vi "InjectionLockServo.vi"() -> ()   [LabVIEW 2020]
panel:
  out "Down times":dbl
  out "Up times":dbl
  out "Currently Output (mA)":dbl
  in  "Initial Output (mA)":dbl
  out "min-max":dbl
  out "min value":dbl
  out "max value":dbl
  in  "?":bool
  in  "Unlock Step\nLength (mA)":dbl
  in  "Semi-lock Step \nLength (mA)":dbl
  in  "Noise Threshold (V)":dbl
  in  "Lock Threshold (V)":dbl
  in  "rate":dbl=10000.0
  in  "milliseconds to wait":u32
  in  "number of samples":i32=100
  out "Waveform Chart":dynamicdata(graph)
  # "Result of Sampling"
  # "Parameters of Feedback"
  # "Parameters of Sampling"
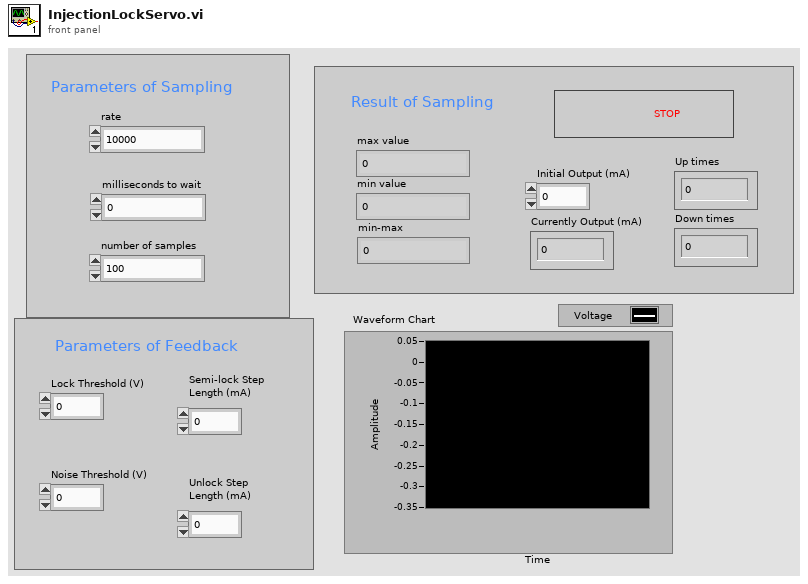
[diagram p1: front panel]
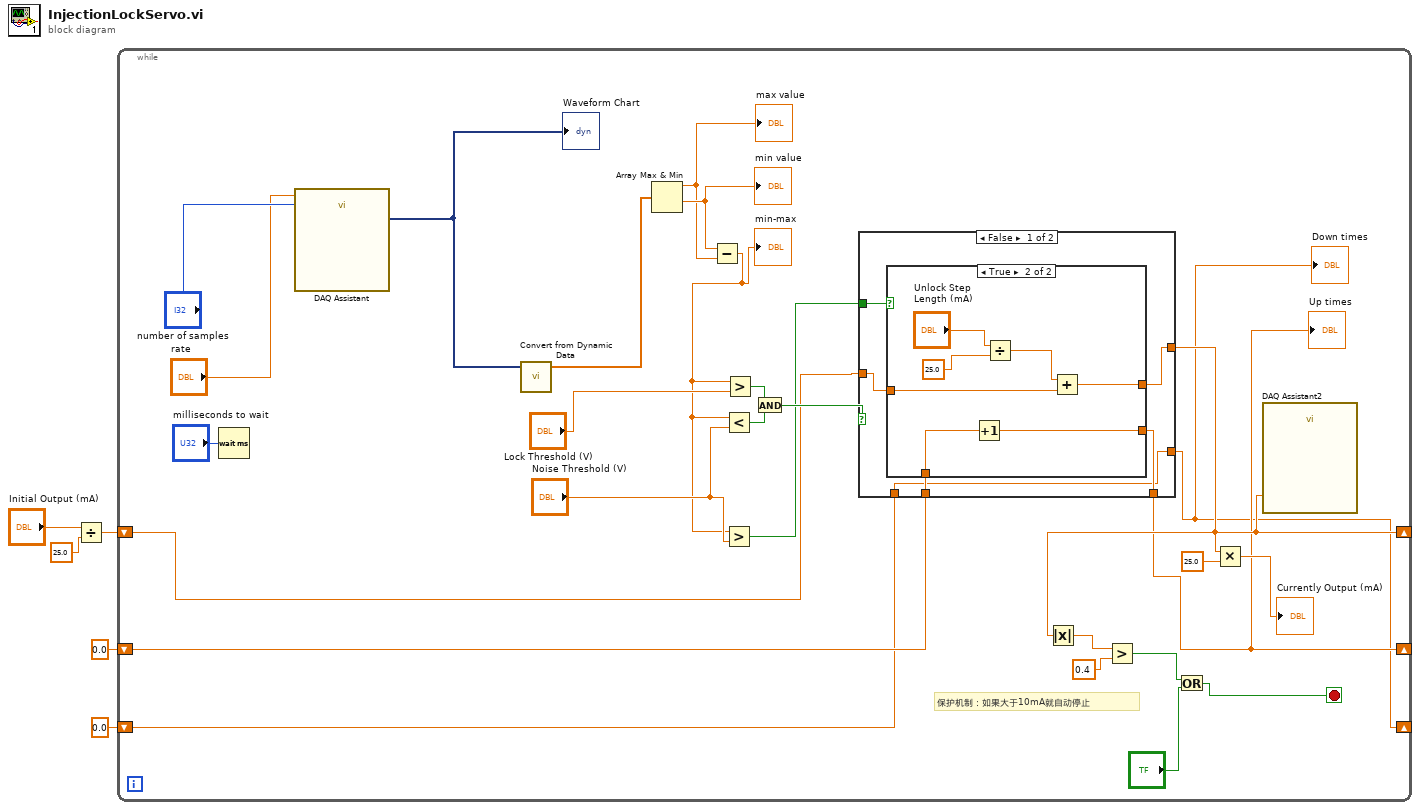
[diagram p0: block diagram]
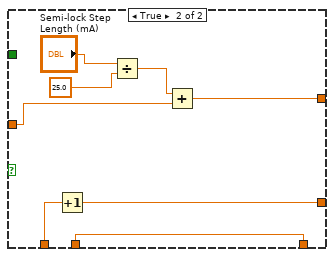
[diagram p3: hidden frame]
diagram:
  n1 = Divide(x="Initial Output (mA)", y=25.0) -> (x/y=w3:dbl)
  n2 = while {
    shift-right: [w13] -> _
    shift-left: w3 -> [w22]
    shift-right: [w10] -> _
    shift-left: 0.0 -> [w12]
    shift-right: [w9] -> _
    shift-left: 0.0 -> [w11]
    stop <- w16 stop-if-true
    # "保护机制：如果大于10mA就自动停止"
    n3 = Wait (ms)(milliseconds to wait="milliseconds to wait") -> ()  [unwired: 1 out]
    n4 = call "DAQ Assistant"("rate"="rate", "number of samples"="number of samples") -> ("data"=w32:dynamicdata)  [unwired: 15 in, 2 out]
    "Waveform Chart" <- w32
    n5 = call "Convert from Dynamic Data"("Dynamic Data Type"=w32) -> ("Array"=w31:dbl[])  [unwired: 3 in]
    n6 = Array Max & Min(array=w31) -> (max value=w7:dbl, min value=w8:dbl)  [unwired: 2 out]
    "max value" <- w7
    "min value" <- w8
    n7 = Subtract(x=w8, y=w7) -> (x-y=w6:dbl)
    "min-max" <- w6
    n8 = Less?(x=w6, y="Noise Threshold (V)") -> (x < y?=w25:bool)
    n9 = Greater?(x=w6, y="Noise Threshold (V)") -> (0:w21:bool)
    n10 = Greater?(x=w6, y="Lock Threshold (V)") -> (0:w26:bool)
    n11 = And(x=w26, y=w25) -> (x .and. y?=w24:bool)
    n12 = case shown="False" w24 {
      tunnel: w22 -> [w37 w52]
      tunnel: [w36 w51] -> w13
      tunnel: w21 -> [w38 _]
      tunnel: w12 -> [w35 w50]
      tunnel: [w34 w50] -> w10
      tunnel: w11 -> [w33 w49]
      tunnel: [w33 w48] -> w9
      frame False {
        n13 = case shown="True" w38 {
          tunnel: w37 -> [w40 w44]
          tunnel: [w40 w43] -> w36
          tunnel: [w39 w42] -> w34
          tunnel: w35 -> [w39 w41]
          frame False {
          }
          frame True {
            n14 = Increment(x=w41) -> (x+1=w42:dbl)
            n15 = Divide(x="Unlock Step\nLength (mA)", y=25.0) -> (x/y=w45:dbl)
            n16 = Add(x=w45, y=w44) -> (x+y=w43:dbl)
          }
        }
      }
      frame True {
        n17 = Increment(x=w49) -> (x+1=w48:dbl)
        n18 = Divide(x="Semi-lock Step \nLength (mA)", y=25.0) -> (x/y=w53:dbl)
        n19 = Add(x=w53, y=w52) -> (x+y=w51:dbl)
      }
    }
    "Up times" <- w10
    "Down times" <- w9
    n20 = Absolute Value(x=w13) -> (abs(x)=w20:dbl)
    n21 = Greater?(x=w20, y=0.4) -> (0:w18:bool)
    n22 = Or(x=w18, y="?") -> (x .or. y?=w16:bool)
    n23 = Multiply(x=w13, y=25.0) -> (x*y=→"Currently Output (mA)":dbl)
    n24 = call "DAQ Assistant2"("data"=w13) -> ()  [unwired: 17 in, 2 out]
  }
